vi "Open Bus Monitor.vi"(8 "error in (no error)":errorcluster, 11 "Mediator in":refnum<class "Mediator.lvclass">) -> (0 "error out":errorcluster, 3 "Mediator out":refnum<class "Mediator.lvclass">)   [LabVIEW 2015, in "Mediator.lvlib" / "Mediator.lvclass"]
uses:
  Mediator.lvclass
  IViewable/IViewable/View Position Enum.ctl
  Mediator.lvclass/Mediator.ctl
  IViewable/IViewable Messages/Open View Msg/Open View Msg.lvclass/Open View Msg.ctl
  <vilib>/ActorFramework/Message Enqueuer/Message Enqueuer.lvclass/Message Enqueuer.ctl
  <vilib>/ActorFramework/Message Enqueuer/Enqueue.vi
  <vilib>/ActorFramework/Message Priority Queue/Priority Enqueue.vi
  IViewable/IViewable Messages/Open View Msg/Open View Msg.lvclass
  IViewable/IViewable/IViewable.lvclass
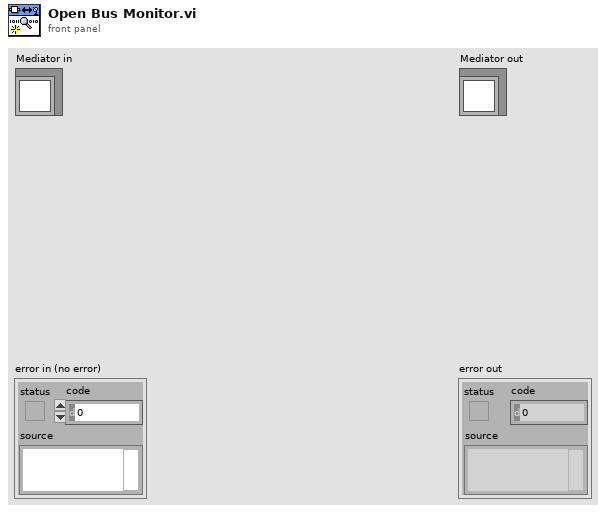
[diagram p1: front panel]
types:
  T1 = typedef "IViewable.lvlib/IViewable.lvclass/View Position Enum.ctl" = enum16{"Centered", "Maximized", "Minimized", "Custom", "Unchanged"}
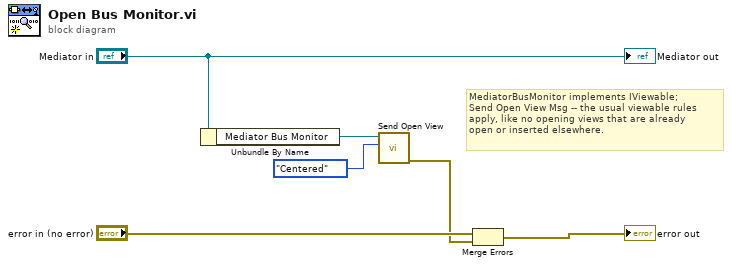
[diagram p0: block diagram]
diagram:
  # "MediatorBusMonitor implements IViewable;\nSend Open View Msg -- the usual viewable rules\napply, like no opening views that are already\nopen or inserted elsewhere."
  n1 = Unbundle By Name("Mediator in") -> ("Mediator Bus Monitor"=w4:refnum<class "Message Enqueuer.lvclass">)
  n2 = call "Send Open View.vi"("Position"=View_Position_Enum."Centered", "Message Enqueuer"=w4) -> ("error out"=w2:errorcluster)  [unwired: 8 in, 1 out]
  n3 = Merge Errors("error in (no error)", w2) -> (→"error out":errorcluster)
  "Mediator out" <- "Mediator in"
